vi "GetEventRefnum.vi"(8 "error in (no error)":errorcluster, 11 "object in":refnum<class "EventMsg.lvclass">) -> (0 "error out":errorcluster, 2 "MsgEvent":refnum<user-event>, 3 "object out":refnum<class "EventMsg.lvclass">)   [LabVIEW 2014, in "EventMsg.lvclass"]
uses:
  EventMsg.lvclass
  EventMsg.lvclass/EventMsg.ctl
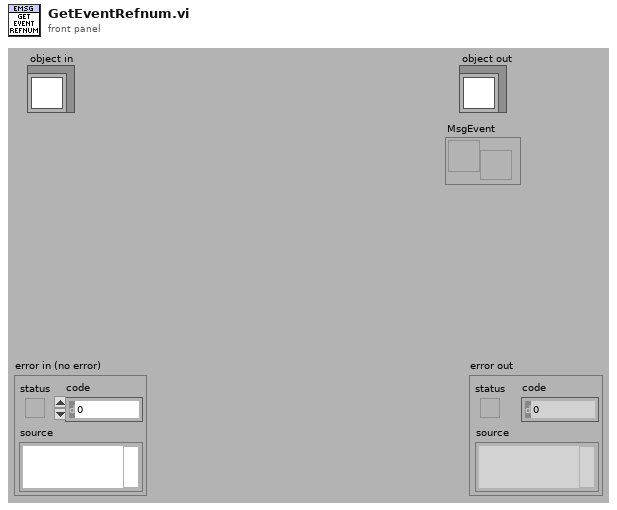
[diagram p1: front panel]
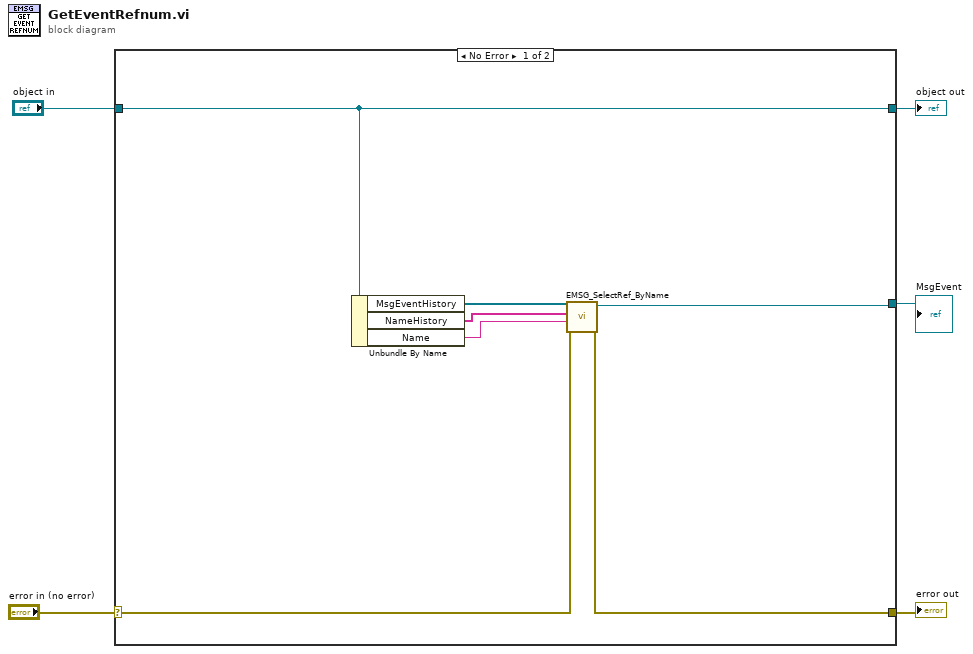
[diagram p0: block diagram]
diagram:
  n1 = case shown="No Error" "error in (no error)" {
    selector: "error in (no error)" -> [w8 w14]
    tunnel: [w7 w14] -> w4
    tunnel: [w12 w13] -> w2
    tunnel: "object in" -> [w12 w13]
    tunnel: [w9 _] -> w1
    frame No Error {
      n2 = Unbundle By Name(w12) -> ("MsgEventHistory"=w11:refnum<user-event>[], "NameHistory"=w10:string[], "Name"=w6:string)
      n3 = call "EMSG_SelectRef_ByName.vi"("Error in"=w8, "Name"=w6, "NameHistory"=w10, "MsgEventHistory"=w11) -> ("Error out"=w7:errorcluster, "User Event out"=w9:refnum<user-event>)  [unwired: 6 in]
    }
    frame Error {
    }
  }
  "error out" <- w4
  "object out" <- w2
  "MsgEvent" <- w1
